vi "Run Pre-Hook.vi"(8 "Error In":errorcluster, 10 "Abstract Syntax Tree In":refnum<class "Root.lvclass">, 11 "Context In":refnum<class "Compiler.lvclass">) -> (0 "Error Out":errorcluster, 2 "Abstract Syntax Tree Out":refnum<class "Root.lvclass">, 3 "Context Out":refnum<class "Compiler.lvclass">)   [LabVIEW 2018, in "Toolkit.lvlib" / "Renderer.lvclass"]
uses:
  Renderer.lvclass
  Hooks/Render/Process/Process.lvclass
  Context/Compiler.lvclass
  Data/Datum/Datum.lvclass
  Nodes/Root/Root.lvclass
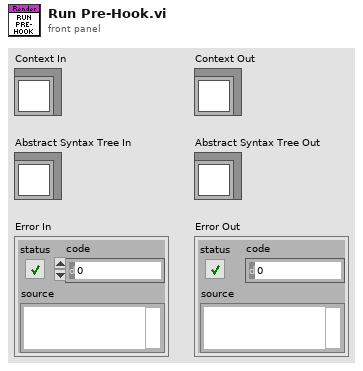
[diagram p1: front panel]
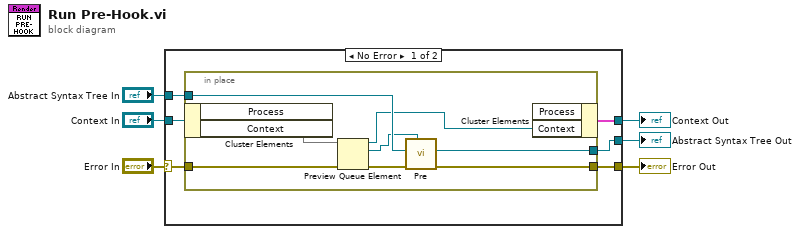
[diagram p0: block diagram]
diagram:
  n1 = case shown="No Error" "Error In" {
    selector: "Error In" -> [w7 w22]
    tunnel: [w12 w23] -> w1
    tunnel: "Context In" -> [w11 w23]
    tunnel: [w10 w21] -> w6
    tunnel: "Abstract Syntax Tree In" -> [w9 w21]
    tunnel: [w8 w22] -> w4
    frame No Error {
      n2 = in-place {
        in-place-border: w7 -> [w20]
        in-place-border: [w19] -> w8
        in-place-border: w9 -> [w18]
        in-place-border: [w17] -> w10
        n3 = in-place-cluster #1(w11) -> ("Context"=w15)  [unwired: 1 out]
        n4 = Preview Queue Element(queue=w15, error in (no error)=w20) -> (queue out=w14:refnum<queue>, element=w13:refnum<class "Datum.lvclass">, error out=w16:errorcluster)  [unwired: 1 in, 1 out]
        n5 = call-dynamic "Pre.vi"("Datum"=w13, "Error In"=w16, "Abstract Syntax Tree In"=w18) -> ("Error Out"=w19:errorcluster, "Abstract Syntax Tree Out"=w17:refnum<class "Root.lvclass">)  [unwired: 6 in, 1 out]
        n6 = in-place-cluster #1("Context"=w14) -> (w12:cluster{})  [unwired: 1 in]
      }
    }
    frame Error {
    }
  }
  "Abstract Syntax Tree Out" <- w6
  "Error Out" <- w4
  "Context Out" <- w1
